vi "IRGetLastCode.vi"(0 "error in (no error)":errorcluster, 3 "Device In":u64) -> (7 "error out":errorcluster, 8 "Bit Count":i32, 9 "Code String":string caption="Code", 10 "Device Out":u64)   [LabVIEW 2012, in "Phidget IR.lvlib"]
doc: "${GetLastCode:Header}"
uses:
  <instrlib>/Phidgets/Phidget IR/Phidget IR.lvlib
  <instrlib>/Phidgets/Phidget Common/Phidget Common.lvlib
  phidget22.dll
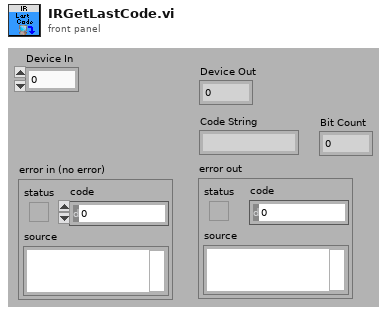
[diagram p1: front panel]
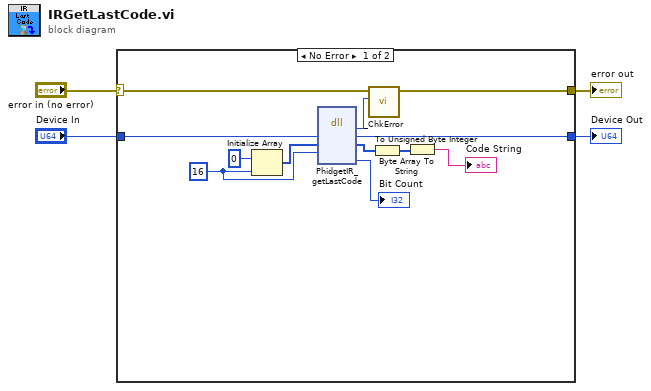
[diagram p0: block diagram]
diagram:
  n1 = case shown="No Error" "error in (no error)" {
    selector: "error in (no error)" -> [w13 w18]
    tunnel: [w12 w18] -> w3
    tunnel: "Device In" -> [w16 w17]
    tunnel: [w15 w17] -> w1
    frame No Error {
      w5 = 16
      n2 = Initialize Array(i8 0, w5) -> (w9:i8[])
      n3 = dll-call lib="phidget22.*" fn="PhidgetIR_getLastCode"("phid"=w16, "codestr"=w9, "codeStrLength"=w5) -> ("return type"=w14:i32, "phid"=w15:u64, "codestr"=w8:i8[], "bitCount"=→"Bit Count":i32)  [unwired: 5 in, 2 out]
      n4 = call <instrlib>:"_ChkError.vi"("Return Code"=w14, "error in (no error)"=w13) -> ("error out"=w12:errorcluster)  [unwired: 9 in]
      n5 = To Unsigned Byte Integer(number=w8) -> (unsigned 8bit integer=w7:u8[])
      n6 = Byte Array To String(unsigned byte array=w7) -> (string=→"Code String":string)
    }
    frame Error {
    }
  }
  "error out" <- w3
  "Device Out" <- w1
